vi "CursorMove.vi"(7 "Enum":T1(ring), 11 "Cursor":cluster{"CursorMin":dbl, "CursorMax":dbl}={"CursorMin"=0.0, "CursorMax"=1.0}) -> (3 "Cursor":cluster{"CursorMin":dbl, "CursorMax":dbl})   [LabVIEW 2012]
uses:
  FullFile.vi
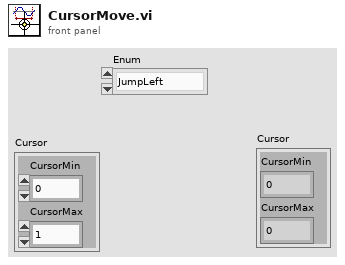
[diagram p1: front panel]
types:
  T1 = enum16{"JumpLeft", "JumpRight", "ScrollLeft", "ScrollRight"}
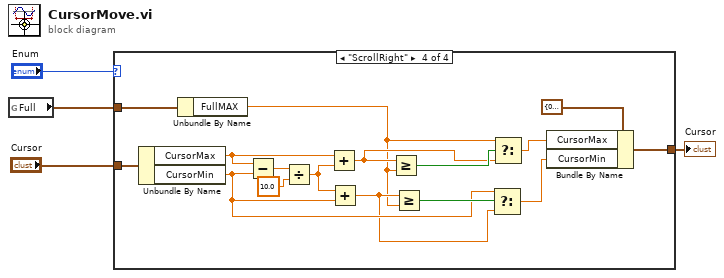
[diagram p0: block diagram]
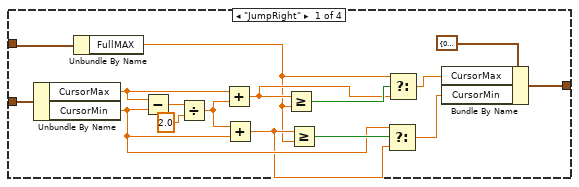
[diagram p2: hidden frame]
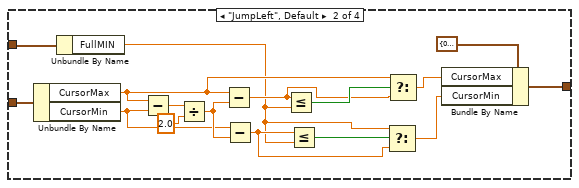
[diagram p3: hidden frame]
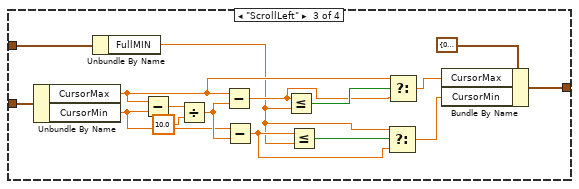
[diagram p4: hidden frame]
diagram:
  n1 = global read "FullFile.vi" "Full"() -> (w1:cluster{"FullMIN":dbl, "FullMAX":dbl})
  n2 = case shown="\"ScrollRight\"" "Enum" {
    tunnel: "Cursor" -> [w18 w34 w50 w66]
    tunnel: w1 -> [w6 w22 w38 w54]
    tunnel: [w7 w26 w42 w55] -> w2
    frame "JumpRight" {
      n3 = Unbundle By Name(w18) -> ("CursorMax"=w10:dbl, "CursorMin"=w15:dbl)
      n4 = Unbundle By Name(w6) -> ("FullMAX"=w5:dbl)
      n5 = Subtract(x=w10, y=w15) -> (x-y=w20:dbl)
      n6 = Divide(x=w20, y=2.0) -> (x/y=w17:dbl)
      n7 = Add(x=w10, y=w17) -> (x+y=w9:dbl)
      n8 = Add(x=w17, y=w15) -> (x+y=w13:dbl)
      n9 = Greater Or Equal?(x=w9, y=w5) -> (x >= y?=w11:bool)
      n10 = Greater Or Equal?(x=w13, y=w5) -> (x >= y?=w16:bool)
      n11 = Select(t=w15, s=w16, f=w13) -> (s? t:f=w12:dbl)
      n12 = Select(t=w5, s=w11, f=w9) -> (s? t:f=w8:dbl)
      n13 = Bundle By Name(cluster=cluster{"CursorMin":dbl, "CursorMax":dbl} {"CursorMin"=0.0, "CursorMax"=0.0} ("输入簇"), "CursorMax"=w8, "CursorMin"=w12) -> (w7:cluster{"CursorMin":dbl, "CursorMax":dbl})
    }
    frame "JumpLeft", Default {
      n14 = Unbundle By Name(w34) -> ("CursorMax"=w24:dbl, "CursorMin"=w31:dbl)
      n15 = Unbundle By Name(w22) -> ("FullMIN"=w21:dbl)
      n16 = Subtract(x=w24, y=w31) -> (x-y=w36:dbl)
      n17 = Divide(x=w36, y=2.0) -> (x/y=w33:dbl)
      n18 = Subtract(x=w24, y=w33) -> (x-y=w23:dbl)
      n19 = Subtract(x=w31, y=w33) -> (x-y=w25:dbl)
      n20 = Less Or Equal?(x=w23, y=w21) -> (x <= y?=w28:bool)
      n21 = Less Or Equal?(x=w25, y=w21) -> (x <= y?=w32:bool)
      n22 = Select(t=w21, s=w32, f=w25) -> (s? t:f=w29:dbl)
      n23 = Select(t=w24, s=w28, f=w23) -> (s? t:f=w27:dbl)
      n24 = Bundle By Name(cluster=cluster{"CursorMin":dbl, "CursorMax":dbl} {"CursorMin"=0.0, "CursorMax"=0.0} ("输入簇"), "CursorMax"=w27, "CursorMin"=w29) -> (w26:cluster{"CursorMin":dbl, "CursorMax":dbl})
    }
    frame "ScrollLeft" {
      n25 = Unbundle By Name(w50) -> ("CursorMax"=w40:dbl, "CursorMin"=w47:dbl)
      n26 = Unbundle By Name(w38) -> ("FullMIN"=w37:dbl)
      n27 = Subtract(x=w40, y=w47) -> (x-y=w52:dbl)
      n28 = Divide(x=w52, y=10.0) -> (x/y=w49:dbl)
      n29 = Subtract(x=w40, y=w49) -> (x-y=w39:dbl)
      n30 = Subtract(x=w47, y=w49) -> (x-y=w41:dbl)
      n31 = Less Or Equal?(x=w39, y=w37) -> (x <= y?=w44:bool)
      n32 = Less Or Equal?(x=w41, y=w37) -> (x <= y?=w48:bool)
      n33 = Select(t=w37, s=w48, f=w41) -> (s? t:f=w45:dbl)
      n34 = Select(t=w40, s=w44, f=w39) -> (s? t:f=w43:dbl)
      n35 = Bundle By Name(cluster=cluster{"CursorMin":dbl, "CursorMax":dbl} {"CursorMin"=0.0, "CursorMax"=0.0} ("输入簇"), "CursorMax"=w43, "CursorMin"=w45) -> (w42:cluster{"CursorMin":dbl, "CursorMax":dbl})
    }
    frame "ScrollRight" {
      n36 = Unbundle By Name(w66) -> ("CursorMax"=w58:dbl, "CursorMin"=w63:dbl)
      n37 = Unbundle By Name(w54) -> ("FullMAX"=w53:dbl)
      n38 = Subtract(x=w58, y=w63) -> (x-y=w68:dbl)
      n39 = Divide(x=w68, y=10.0) -> (x/y=w65:dbl)
      n40 = Add(x=w58, y=w65) -> (x+y=w57:dbl)
      n41 = Add(x=w65, y=w63) -> (x+y=w61:dbl)
      n42 = Greater Or Equal?(x=w57, y=w53) -> (x >= y?=w59:bool)
      n43 = Greater Or Equal?(x=w61, y=w53) -> (x >= y?=w64:bool)
      n44 = Select(t=w63, s=w64, f=w61) -> (s? t:f=w60:dbl)
      n45 = Select(t=w53, s=w59, f=w57) -> (s? t:f=w56:dbl)
      n46 = Bundle By Name(cluster=cluster{"CursorMin":dbl, "CursorMax":dbl} {"CursorMin"=0.0, "CursorMax"=0.0} ("输入簇"), "CursorMax"=w56, "CursorMin"=w60) -> (w55:cluster{"CursorMin":dbl, "CursorMax":dbl})
    }
  }
  "Cursor" <- w2
